vi "Drive PID.vi"(7 "Description":string, 8 "Command Info In":T1, 9 "Speed":dbl, 10 "Distance":dbl, 11 "Target Angle":dbl) -> (0 "Command Info Out":T1)   [LabVIEW 2017]
doc: "This VI notifies the subsystem to perform this command for the given duration, then go back to the default state. Synchronization determines whether this VI Starts the operation and returns immediately, or waits for the operation to complete. The first option is commonly used for TeleOp, and the second for Autonomous sequencing."
uses:
  <vilib>/Rock Robotics/WPI/Framework/Command Status Info.ctl
  <vilib>/Rock Robotics/WPI/Framework/Completion Status.ctl
  <vilib>/Rock Robotics/WPI/Framework/Completion Notifier.ctl
  Implementation/Drive Setpoints.ctl
  Implementation/Drive Operations.ctl
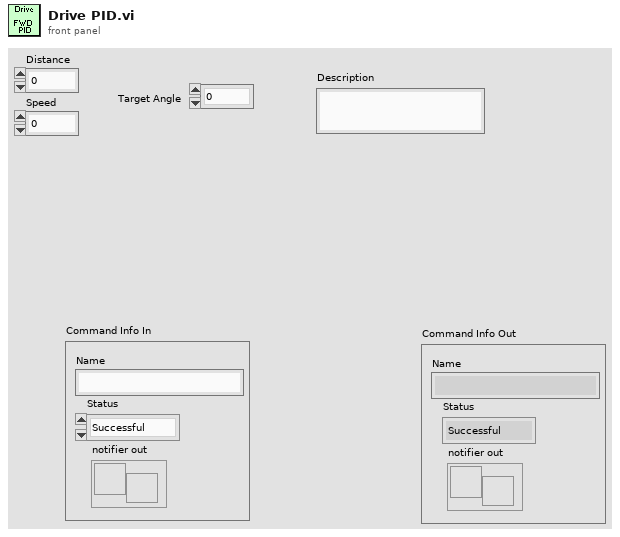
[diagram p1: front panel]
types:
  T1 = typedef "Command Status Info.ctl" = cluster{"Name":string, "Status":T2, "notifier out":T3}
  T2 = typedef "Completion Status.ctl" = enum16{"Successful", "Aborted", "Incomplete"}
  T3 = typedef "Completion Notifier.ctl" = refnum<notifier>
  T4 = typedef "Drive Setpoints.ctl" = cluster{"Operation":T5, "Left Setpoint":dbl, "Right Setpoint":dbl, "Duration":dbl, "Distance":dbl, "Target Angle":dbl, "Speed":dbl}
  T5 = typedef "Drive Operations.ctl" = enum16{"Reserve", "Read Current", "Immediate", "Drive for Time", "Drive for Distance", "Drive PID", "Auto Turn", "Reset Encoders", "Reset Gyro"}
  T6 = typedef "WPI_EncoderDevRef.ctl" = cluster{"DevStatus":errorcluster, "EncoderIndex":T7, "CounterIndex":T8, "DistancePerCount":dbl, "Decoding Type":T9}
  T7 = typedef "FPGA_EncoderIdx.ctl" = enum8{"Enc 0", "Enc 1", "Enc 2", "Enc 3", "Enc 4", "Enc 5", "Enc 6", "Enc 7", "Invalid"}
  T8 = typedef "FPGA_CounterCtrSystemIndex.ctl" = enum8{"Ctr 0", "Ctr 1", "Ctr 2", "Ctr 3", "Ctr 4", "Ctr 5", "Ctr 6", "Ctr 7", "Invalid"}
  T9 = typedef "WPI_EncoderType.ctl" = enum16{"1x", "2x", "4x"}
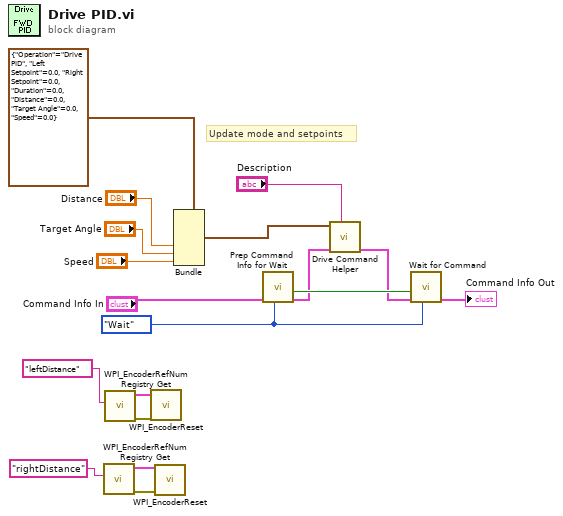
[diagram p0: block diagram]
diagram:
  w10 = enum16{"Start", "Wait"}."Wait" ("Synchronication")
  # "Update mode and setpoints"
  n1 = call <vilib>:"WPI_EncoderRefNum Registry Get.vi"("refnum name"="rightDistance") -> ("error out"=w1:errorcluster, "EncoderDevRef"=w2:T6)  [unwired: 9 in]
  n2 = call <vilib>:"WPI_EncoderRefNum Registry Get.vi"("refnum name"="leftDistance") -> ("error out"=w4:errorcluster, "EncoderDevRef"=w3:T6)  [unwired: 9 in]
  n3 = call <vilib>:"WPI_EncoderReset.vi"("error in (no error)"=w4, "EncoderDevRef"=w3) -> ()  [unwired: 8 in, 2 out]
  n4 = call <vilib>:"WPI_EncoderReset.vi"("error in (no error)"=w1, "EncoderDevRef"=w2) -> ()  [unwired: 8 in, 2 out]
  n5 = Bundle(cluster=T4 {"Operation"=enum."Drive PID", "Left Setpoint"=0.0, "Right Setpoint"=0.0, "Duration"=0.0, "Distance"=0.0, "Target Angle"=0.0, "Speed"=0.0} ("SubSystem Data"), "Distance"="Distance", "Target Angle"="Target Angle", "Speed"="Speed") -> (w11:T4)  [unwired: 4 in]
  n6 = call <vilib>:"Prep Command Info for Wait.vi"("Synchronication"=w10, "Command Info"="Command Info In") -> ("Command Info"=w15:T1, "Allocated"=w16:bool)  [unwired: 8 in]
  n7 = call "Drive Command Helper.vi"("Description"="Description", "Command Info In"=w15, "SubSystem Data"=w11) -> ("Command Info Out"=w12:T1)  [unwired: 6 in, 2 out]
  n8 = call <vilib>:"Wait for Command.vi"("Synchronication"=w10, "Command Info in"=w12, "Allocated"=w16) -> ("Command Info out"=→"Command Info Out":T1)  [unwired: 8 in]
